vi "LWXPS_PositionerHardwareStatusStringGet.vi"(0 "XPS Reference IN":refnum<k24>, 7 "Positioner hardware status":i32, 11 "LabVIEW error IN":errorcluster) -> (4 "XPS Reference OUT":refnum<k24>, 6 "Returned error code":i32, 8 "Positioner hardware status description":string, 10 "XPS Error String":string, 15 "LabVIEW error OUT":errorcluster)   [LabVIEW 2014]
uses:
  D:/XPSQ8_LabView_Library/Development/Source/Dll/Newport.XPS.CommandInterface.dll
  Dll/Newport.XPS.CommandInterface.dll
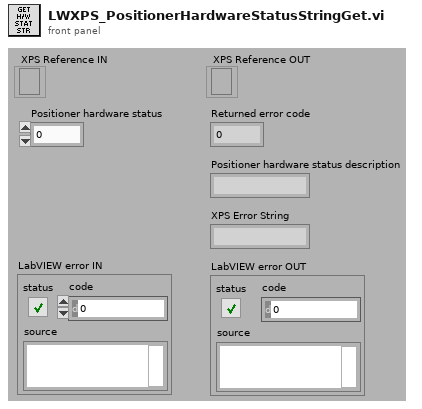
[diagram p1: front panel]
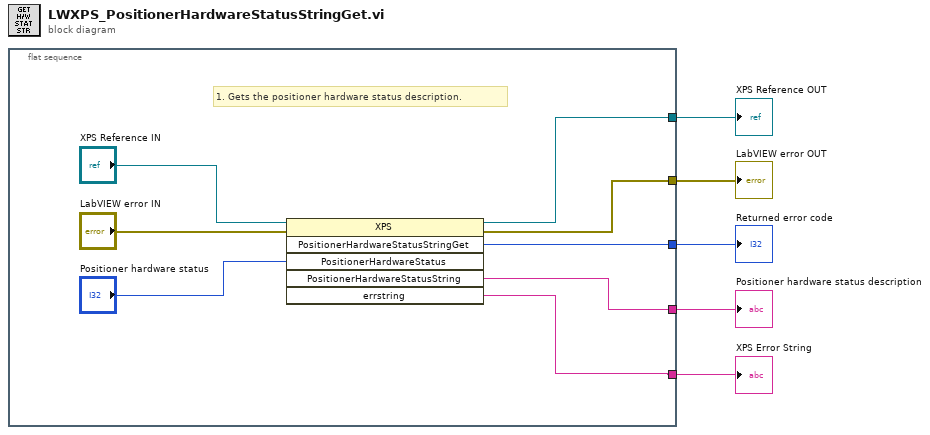
[diagram p0: block diagram]
diagram:
  n1 = flat-sequence {
    tunnel: [w11] -> w5
    tunnel: [w9] -> w4
    tunnel: [w12] -> w3
    tunnel: [w6] -> w1
    tunnel: [w7] -> w2
    frame #0 {
      # "1. Gets the positioner hardware status description."
      n2 = invoke class="XPS" method="PositionerHardwareStatusStringGet"(reference="XPS Reference IN", error in="LabVIEW error IN", "PositionerHardwareStatus"="Positioner hardware status") -> (reference out=w11:refnum<k24>, error out=w9:errorcluster, "PositionerHardwareStatusStringGet"=w12:i32, "PositionerHardwareStatusString"=w7:string, "errstring"=w6:string)  [unwired: 3 in, 1 out]
    }
  }
  "XPS Error String" <- w1
  "XPS Reference OUT" <- w5
  "LabVIEW error OUT" <- w4
  "Returned error code" <- w3
  "Positioner hardware status description" <- w2
